vi "VI Scripting Create Path From Template.vi"(5 "Graph":cluster{dbl[], dbl[]}[](array[cluster]), 6 "VI in":refnum<vi>, 7 "Name":string, 9 "path":cluster{"X":dbl, "Y":dbl}[](array[cluster]), 10 "Data Points":T1[](array[typedef]), 11 "base path":path) -> ()   [LabVIEW 2018]
uses:
  Typedef/Data Point.ctl
  <vilib>/LabVIEW Icon API/API_Rectangle Dimension.ctl
  <vilib>/LabVIEW Icon API/API_Text.ctl
  <vilib>/LabVIEW Icon API/LabVIEW Icon API.lvlib
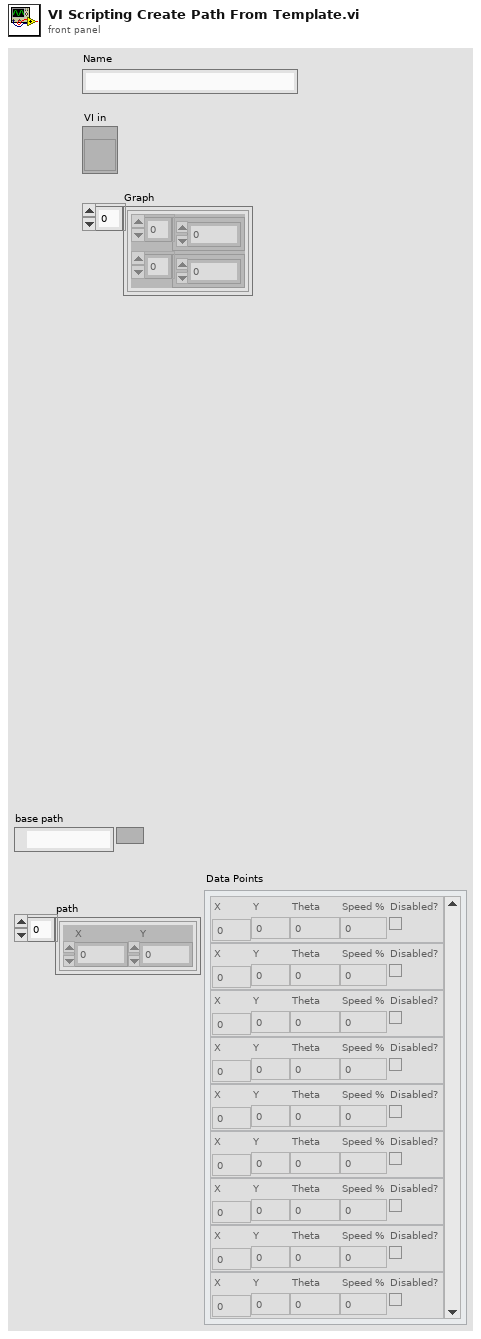
[diagram p1: front panel]
types:
  T1 = typedef "Data Point.ctl" = cluster{"X":dbl, "Y":dbl, "Theta":dbl, "Speed %":dbl, "Disabled?":bool}
  T2 = typedef "LabVIEW Icon API.lvlib/API_Text.ctl" = cluster{"Line 1 text":string, "Line 2 text":string, "Line 3 text":string, "Line 4 text":string}
  T3 = typedef "LabVIEW Icon API.lvlib/API_Rectangle Dimension.ctl" = cluster{"Width":i16, "Height":i16}
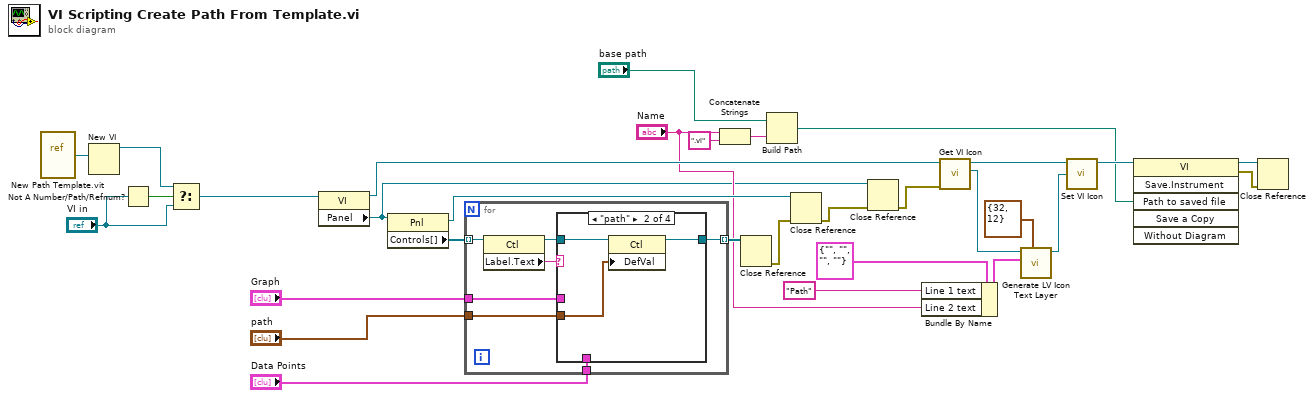
[diagram p0: block diagram]
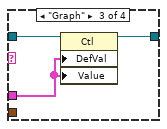
[diagram p3: hidden frame]
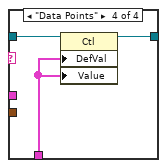
[diagram p4: hidden frame]
diagram:
  n1 = vi-ref "New Path Template.vit"() -> (w9:refnum<vi>)
  n2 = New VI(10:w9) -> (3:w11:refnum<vi>)  [unwired: 6 in, 1 out]
  n3 = Not A Number/Path/Refnum?(number/path/refnum="VI in") -> (NaN/Path/Refnum?=w8:bool)
  n4 = Select(t=w11, s=w8, f="VI in") -> (s? t:f=w10:refnum<vi>)
  n5 = property class="VI"(reference=w10) -> (reference out=w31:refnum<vi>, "Panel"=w14:refnum<vi>)  [unwired: 1 in, 1 out]
  n6 = property class="Pnl"(reference=w14) -> (reference out=w21:refnum<vi>, "Controls[]"=w17:refnum<vi>[])  [unwired: 1 in, 1 out]
  n7 = for {
    tunnel: w17 -> [w38] mode=indexing
    tunnel: "Graph" -> [w35]
    tunnel: [w34] -> w19 mode=indexing
    tunnel: "path" -> [w33]
    tunnel: "Data Points" -> [w32]
    n8 = property class="Ctl"(reference=w38) -> (reference out=w36:refnum<vi>, "Label.Text"=w37:string)  [unwired: 1 in, 1 out]
    n9 = case shown="\"path\"" w37 {
      tunnel: w36 -> [w39 w42 w45 w48]
      tunnel: w35 -> [_ _ w43 _]
      tunnel: [w39 w41 w44 w47] -> w34
      tunnel: w33 -> [_ w40 _ _]
      tunnel: w32 -> [_ _ _ w46]
      frame Default {
      }
      frame "path" {
        n10 = property class="Ctl"(reference=w42, "DefVal"=w40) -> (reference out=w41:refnum<vi>)  [unwired: 1 in, 1 out]
      }
      frame "Graph" {
        n11 = property class="Ctl"(reference=w45, "DefVal"=w43, "Value"=w43) -> (reference out=w44:refnum<vi>)  [unwired: 1 in, 1 out]
      }
      frame "Data Points" {
        n12 = property class="Ctl"(reference=w48, "DefVal"=w46, "Value"=w46) -> (reference out=w47:refnum<vi>)  [unwired: 1 in, 1 out]
      }
    }
  }
  n13 = Concatenate Strings("Name", ".vi" ("string")) -> (w22:string)
  n14 = Close Reference(reference=w19) -> (error out=w20:errorcluster)  [unwired: 1 in]
  n15 = Build Path(base path="base path", name or relative path=w22) -> (appended path=w5:path)
  n16 = Close Reference(reference=w21, error in (no error)=w20) -> (error out=w15:errorcluster)
  n17 = Close Reference(reference=w14, error in (no error)=w15) -> (error out=w13:errorcluster)
  n18 = Bundle By Name(cluster=T2 {"Line 1 text"="", "Line 2 text"="", "Line 3 text"="", "Line 4 text"=""} ("Text"), "Line 1 text"="Path", "Line 2 text"="Name") -> (w29:T2)
  n19 = call <vilib>:"Get VI Icon.vi"("error in (no error)"=w13, "VI Refnum in"=w31) -> ("Icon"=w25:refnum<class "Icon.lvclass">, "VI Refnum out"=w24:refnum<vi>)  [unwired: 7 in, 1 out]
  n20 = call <vilib>:"Generate LV Icon Text Layer.vi"("Rectangle dimension (32,32)"=T3 {"Width"=32, "Height"=12}, "Text"=w29, "Icon in"=w25) -> ("Icon out"=w26:refnum<class "Icon.lvclass">)  [unwired: 7 in, 1 out]
  n21 = call <vilib>:"Set VI Icon.vi"("Icon"=w26, "VI Refnum in"=w24) -> ("VI Refnum out"=w6:refnum<vi>)  [unwired: 8 in, 1 out]
  n22 = invoke class="VI" method="Save.Instrument"(reference=w6, "Path to saved file"=w5) -> (reference out=w7:refnum<vi>, error out=w2:errorcluster)  [unwired: 4 in, 4 out]
  n23 = Close Reference(reference=w7, error in (no error)=w2) -> ()  [unwired: 1 out]
